vi "Add VI to lib.vi"(11 "error in":errorcluster) -> (15 "error out":errorcluster)   [LabVIEW 2021, in "Converter.lvlib"]
uses:
  Converter.lvlib
  Converter Reusables/Converter Reusables.lvlib
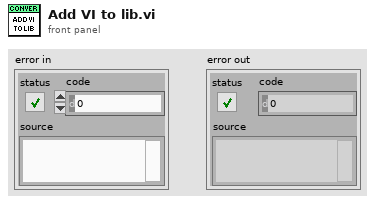
[diagram p1: front panel]
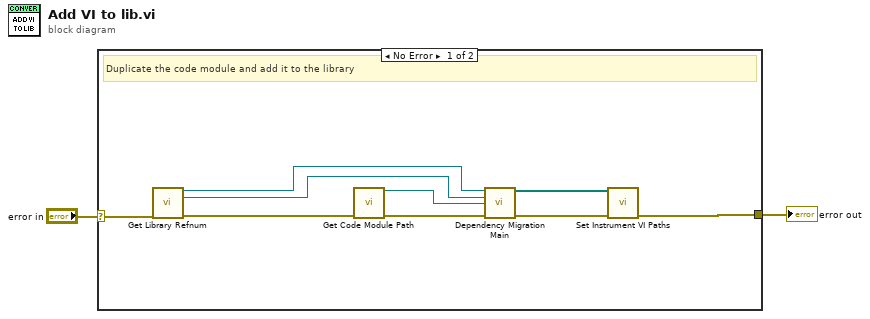
[diagram p0: block diagram]
diagram:
  n1 = case shown="No Error" "error in" {
    selector: "error in" -> [w7 w12]
    tunnel: [w10 w12] -> w1
    frame No Error {
      # "Duplicate the code module and add it to the library"
      n2 = call "Get Library Refnum.vi"("error in (no error)"=w7) -> ("Library Refnum"=w8:refnum<vi>, "Project:Open"=w9:refnum<vi>, "error out"=w11:errorcluster)  [unwired: 12 in]
      n3 = call "Get Code Module Path.vi"("error in (no error)"=w11) -> ("CodeModule Out"=w3:path, "error out"=w6:errorcluster)  [unwired: 13 in]
      n4 = call "Dependency Migration Main.vi"("LibraryRefnum"=w8, "Project:Open"=w9, "SourceModulePath"=w3, "error in (no error)"=w6) -> ("InstrContaining"=w4:path[], "error out"=w5:errorcluster)  [unwired: 10 in]
      n5 = call "Set Instrument VI Paths.vi"("error in (no error)"=w5, "VI Paths[]"=w4) -> ("error out"=w10:errorcluster)  [unwired: 9 in]
    }
    frame Error {
    }
  }
  "error out" <- w1
